vi "Get Platform.vi"(8 "error in (no error)":errorcluster, 11 "Device in":refnum<class "Device.lvclass">) -> (0 "error out":errorcluster, 2 "Platform":refnum<class "Platform.lvclass">, 3 "Device out":refnum<class "Device.lvclass">)   [LabVIEW 2020, in "PicoG-App.lvlib" / "Device.lvclass"]
uses:
  Device.lvclass
  Builds/picoG/ppl/PicoG-Core.lvlibp/PicoG-Processor/PicoG-Core/PlatformManager/PlatformManager.lvclass
  Builds/picoG/ppl/PicoG-Core.lvlibp/PicoG-Processor/PicoG-Core/Platform/Platform.lvclass
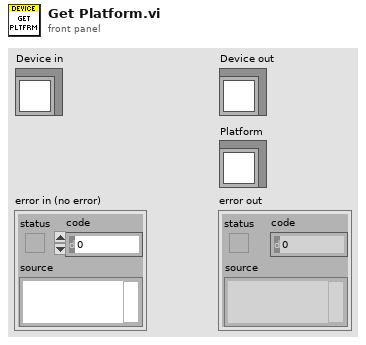
[diagram p1: front panel]
types:
  T1 = typedef "PicoG-App.lvlib/Device.lvclass/Ref Data.ctl" = cluster{"Alias":string, "Version":string, "Build":timestamp, "Key":T2}
  T2 = typedef "PicoG-App.lvlib/Device.lvclass/Device Key.ctl" = cluster{"Platform":string, "Board":string, "ID":string}
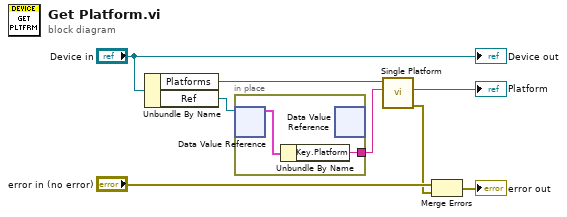
[diagram p0: block diagram]
diagram:
  n1 = Unbundle By Name("Device in") -> ("Platforms"=w4:refnum<class "PlatformManager.lvclass">, "Ref"=w7:refnum<data-value>)
  n2 = in-place {
    in-place-border: [w9] -> w5
    n3 = in-place-dvr #1(w7) -> (w10:T1)  [unwired: 1 out]
    n4 = Unbundle By Name(w10) -> ("Key.Platform"=w9:string)
    n5 = in-place-dvr #1() -> ()  [unwired: 1 in, 2 out]
  }
  n6 = call "Single Platform.vi"("Platform Name"=w5, "PlatformManager in"=w4) -> ("error out"=w1:errorcluster, "Platform"=→"Platform":refnum<class "Platform.lvclass">)  [unwired: 7 in, 1 out]
  n7 = Merge Errors("error in (no error)", w1) -> (→"error out":errorcluster)
  "Device out" <- "Device in"
